vi "LogSum.vi"(11 "Array":dbl[](array[numeric])) -> (3 "Numeric":dbl)   [LabVIEW 2017]
uses:
  <vilib>/Analysis/NI_AALBLAS.lvlib
  <vilib>/Analysis/BLAS.llb/dasum - Absolute Values Sum (DBL).vi
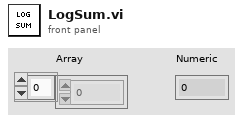
[diagram p1: front panel]
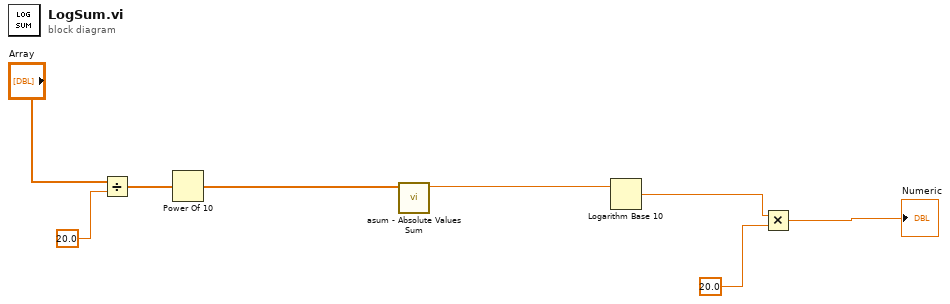
[diagram p0: block diagram]
diagram:
  n1 = Divide(x="Array", y=20.0) -> (x/y=w2:dbl[])
  n2 = Power Of 10(x=w2) -> (10^x=w4:dbl[])
  n3 = call-poly <vilib>:"asum - Absolute Values Sum.vi"("x"=w4) -> ("dasum"=w5:dbl)  [unwired: 9 in, 1 out]
  n4 = Logarithm Base 10(1:w5) -> (0:w7:dbl)
  n5 = Multiply(x=w7, y=20.0) -> (x*y=→"Numeric":dbl)
